vi "Init lib MPSSE.vi"(8 "error in (no error)":errorcluster) -> (0 "error out":errorcluster)   [LabVIEW 2024, in "libMPSSE-I2C.lvlib"]
doc: "FTDI_API void Init_libMPSSE(void);"
uses:
  libMPSSE-I2C.lvlib
  libmpsse.dll
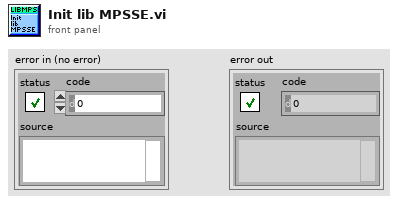
[diagram p1: front panel]
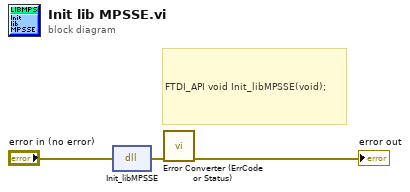
[diagram p0: block diagram]
diagram:
  # "FTDI_API void Init_libMPSSE(void);"
  n1 = dll-call lib="C:/Sandbox/sm_6576_001_RIB_Sequencer/I2C/libmpsse.dll" fn="Init_libMPSSE"(error in="error in (no error)") -> (error out=w1:errorcluster)  [unwired: 3 in, 1 out]
  n2 = call "Error Converter (ErrCode or Status).vi"("error in (no error)"=w1) -> ("error out"=→"error out":errorcluster)  [unwired: 10 in]
